vi "Substitute Layer.vi"(6 "Substitute Layer":refnum<class "Layer.lvclass">, 11 "All User Layers in":refnum<class "Layer.lvclass">[](array[class])) -> (3 "All User Layers out":refnum<class "Layer.lvclass">[](array[class]))   [LabVIEW 2021, in "Layer.lvclass"]
doc: "Substiture a User Layer by Name. If All User Layers in contains a matching Layer Name, it will get substituted with the Substitute User Layer."
uses:
  <vilib>/LabVIEW Icon API/lv_icon/Classes/Layer/Layer.lvclass
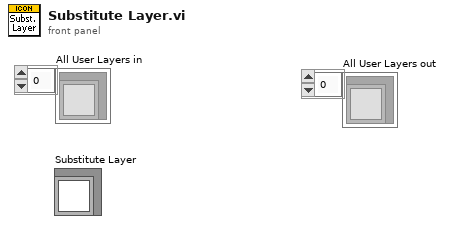
[diagram p1: front panel]
types:
  T1 = typedef "Layer.ctl" = cluster{"LayerIcon":picture, "LayerName":string, "Opacity":u8, "Visibility?":bool}
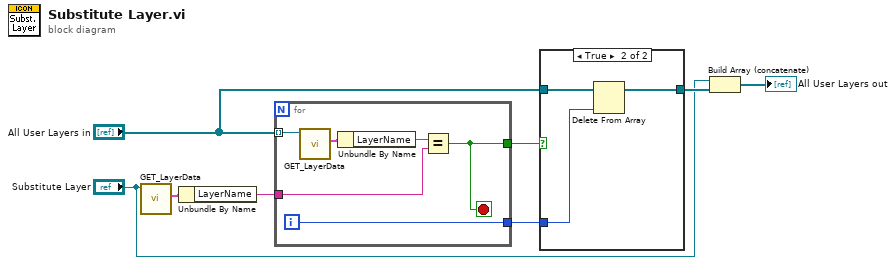
[diagram p0: block diagram]
diagram:
  n1 = call-dynamic "GET_LayerData.vi"("Layer.lvclass in"="Substitute Layer") -> ("Data"=w8:T1)  [unwired: 6 in, 4 out]
  n2 = Unbundle By Name(w8) -> ("LayerName"=w7:string)
  n3 = for {
    tunnel: "All User Layers in" -> [w14] mode=indexing
    tunnel: w7 -> [w11]
    tunnel: [w10] -> w6
    tunnel: [w9] -> w4
    i -> [w9]
    stop <- w10 stop-if-true
    n4 = call-dynamic "GET_LayerData.vi"("Layer.lvclass in"=w14) -> ("Data"=w13:T1)  [unwired: 6 in, 4 out]
    n5 = Unbundle By Name(w13) -> ("LayerName"=w12:string)
    n6 = Equal?(x=w12, y=w11) -> (x = y?=w10:bool)
  }
  n7 = case shown="True" w6 {
    tunnel: "All User Layers in" -> [w15 w18]
    tunnel: w4 -> [_ w17]
    tunnel: [w15 w16] -> w3
    frame False {
    }
    frame True {
      n8 = Delete From Array(array=w18, index=w17) -> (array with subset deleted=w16:refnum<class "Layer.lvclass">[])  [unwired: 1 in, 1 out]
    }
  }
  n9 = Build Array (concatenate)("Substitute Layer", w3) -> (→"All User Layers out":refnum<class "Layer.lvclass">[])
